vi "ToolScanTest.vi"(8 "error in (no error)":errorcluster, 11 "VISA resource name":refnum<visa-resource-name>="COM5") -> (0 "error out":errorcluster, 1 "read string 3":string, 2 "read string 2":string, 3 "read string":string, 4 "read string 6":string, 5 "Array":string[](array[string]))   [LabVIEW 2019]
panel:
  out "read string 13":string
  out "read string 12":string
  out "read string 11":string
  out "read string 10":string
  out "read string 9":string
  out "read string 8":string
  out "read string 5":string
  out "read string 4":string
  in  "stop":bool
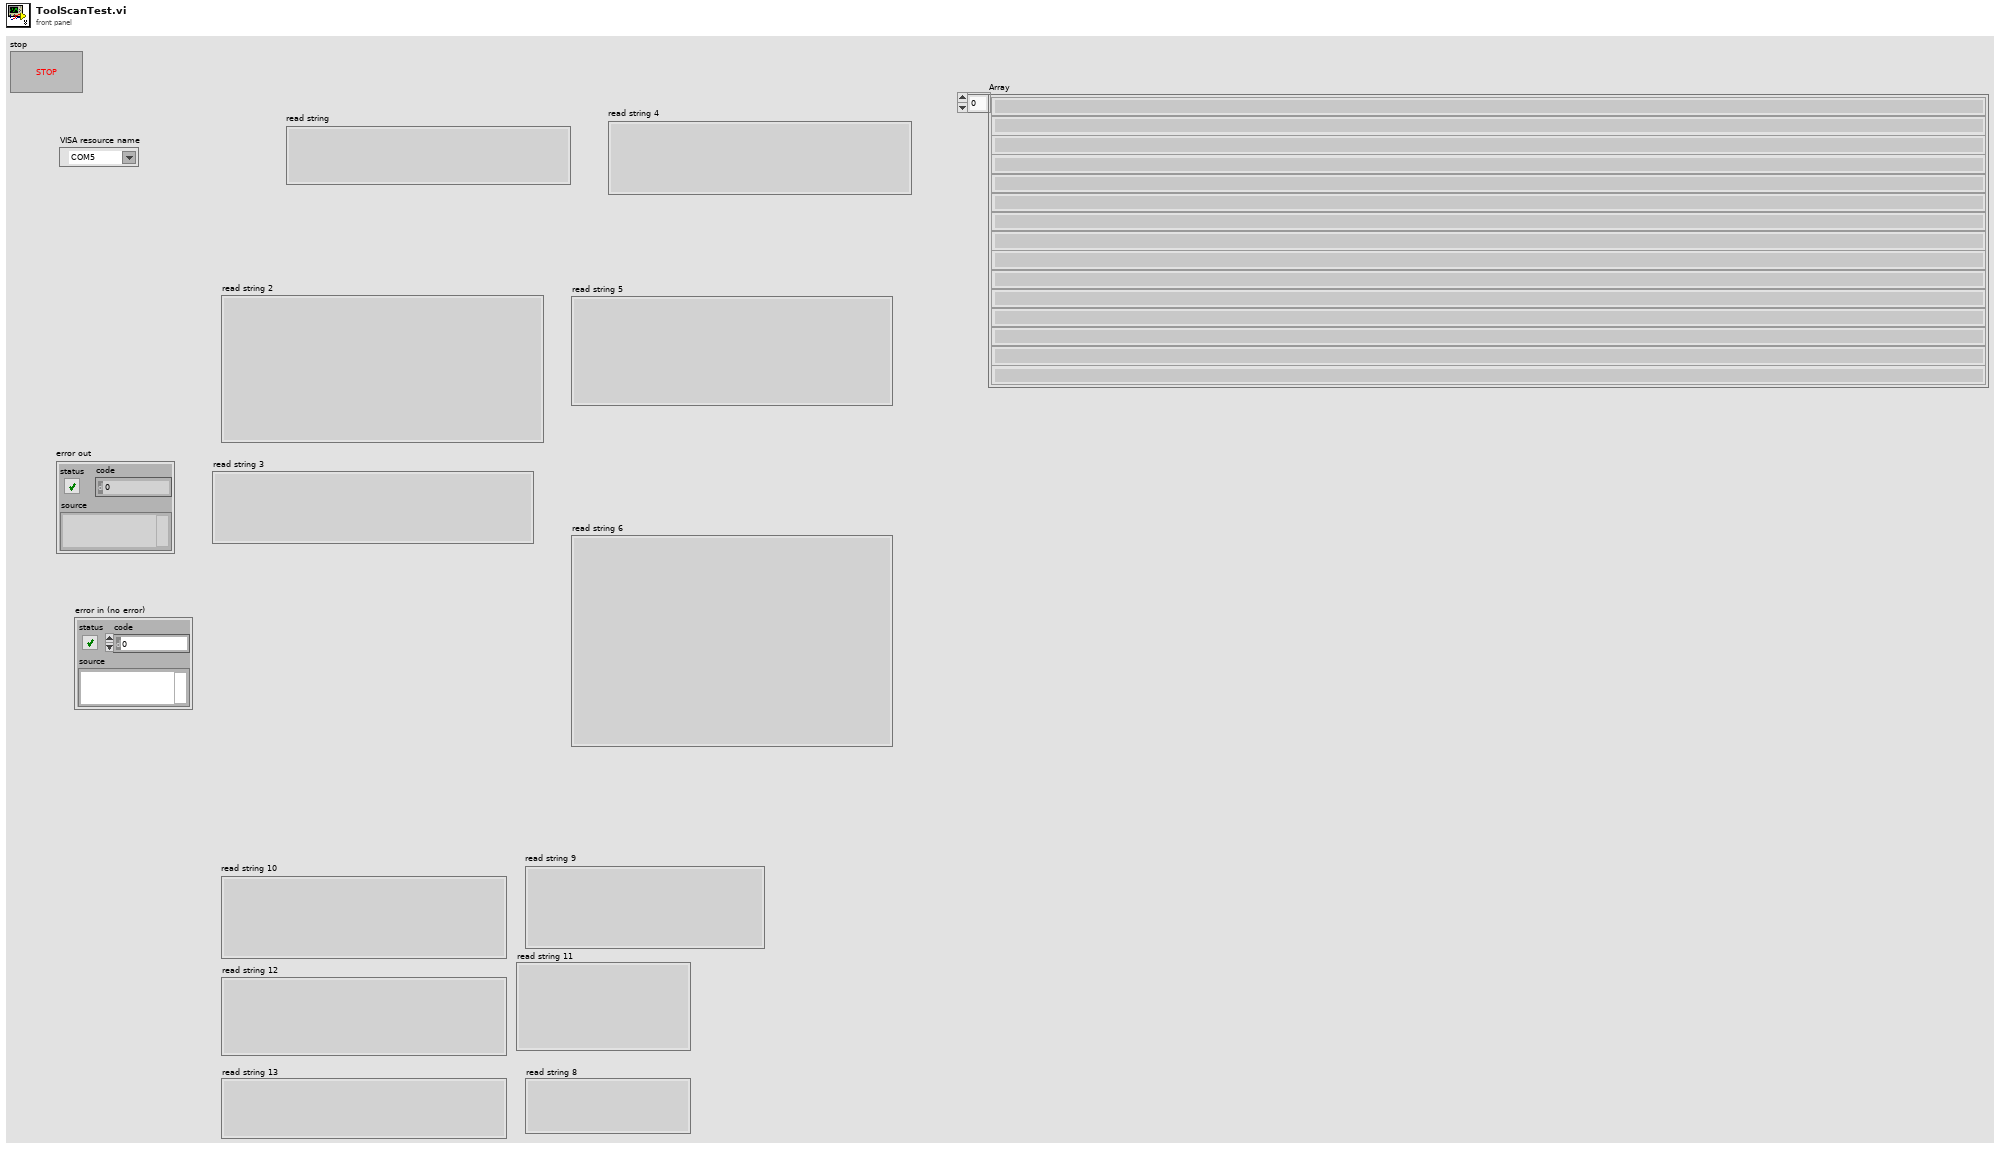
[diagram p1: front panel]
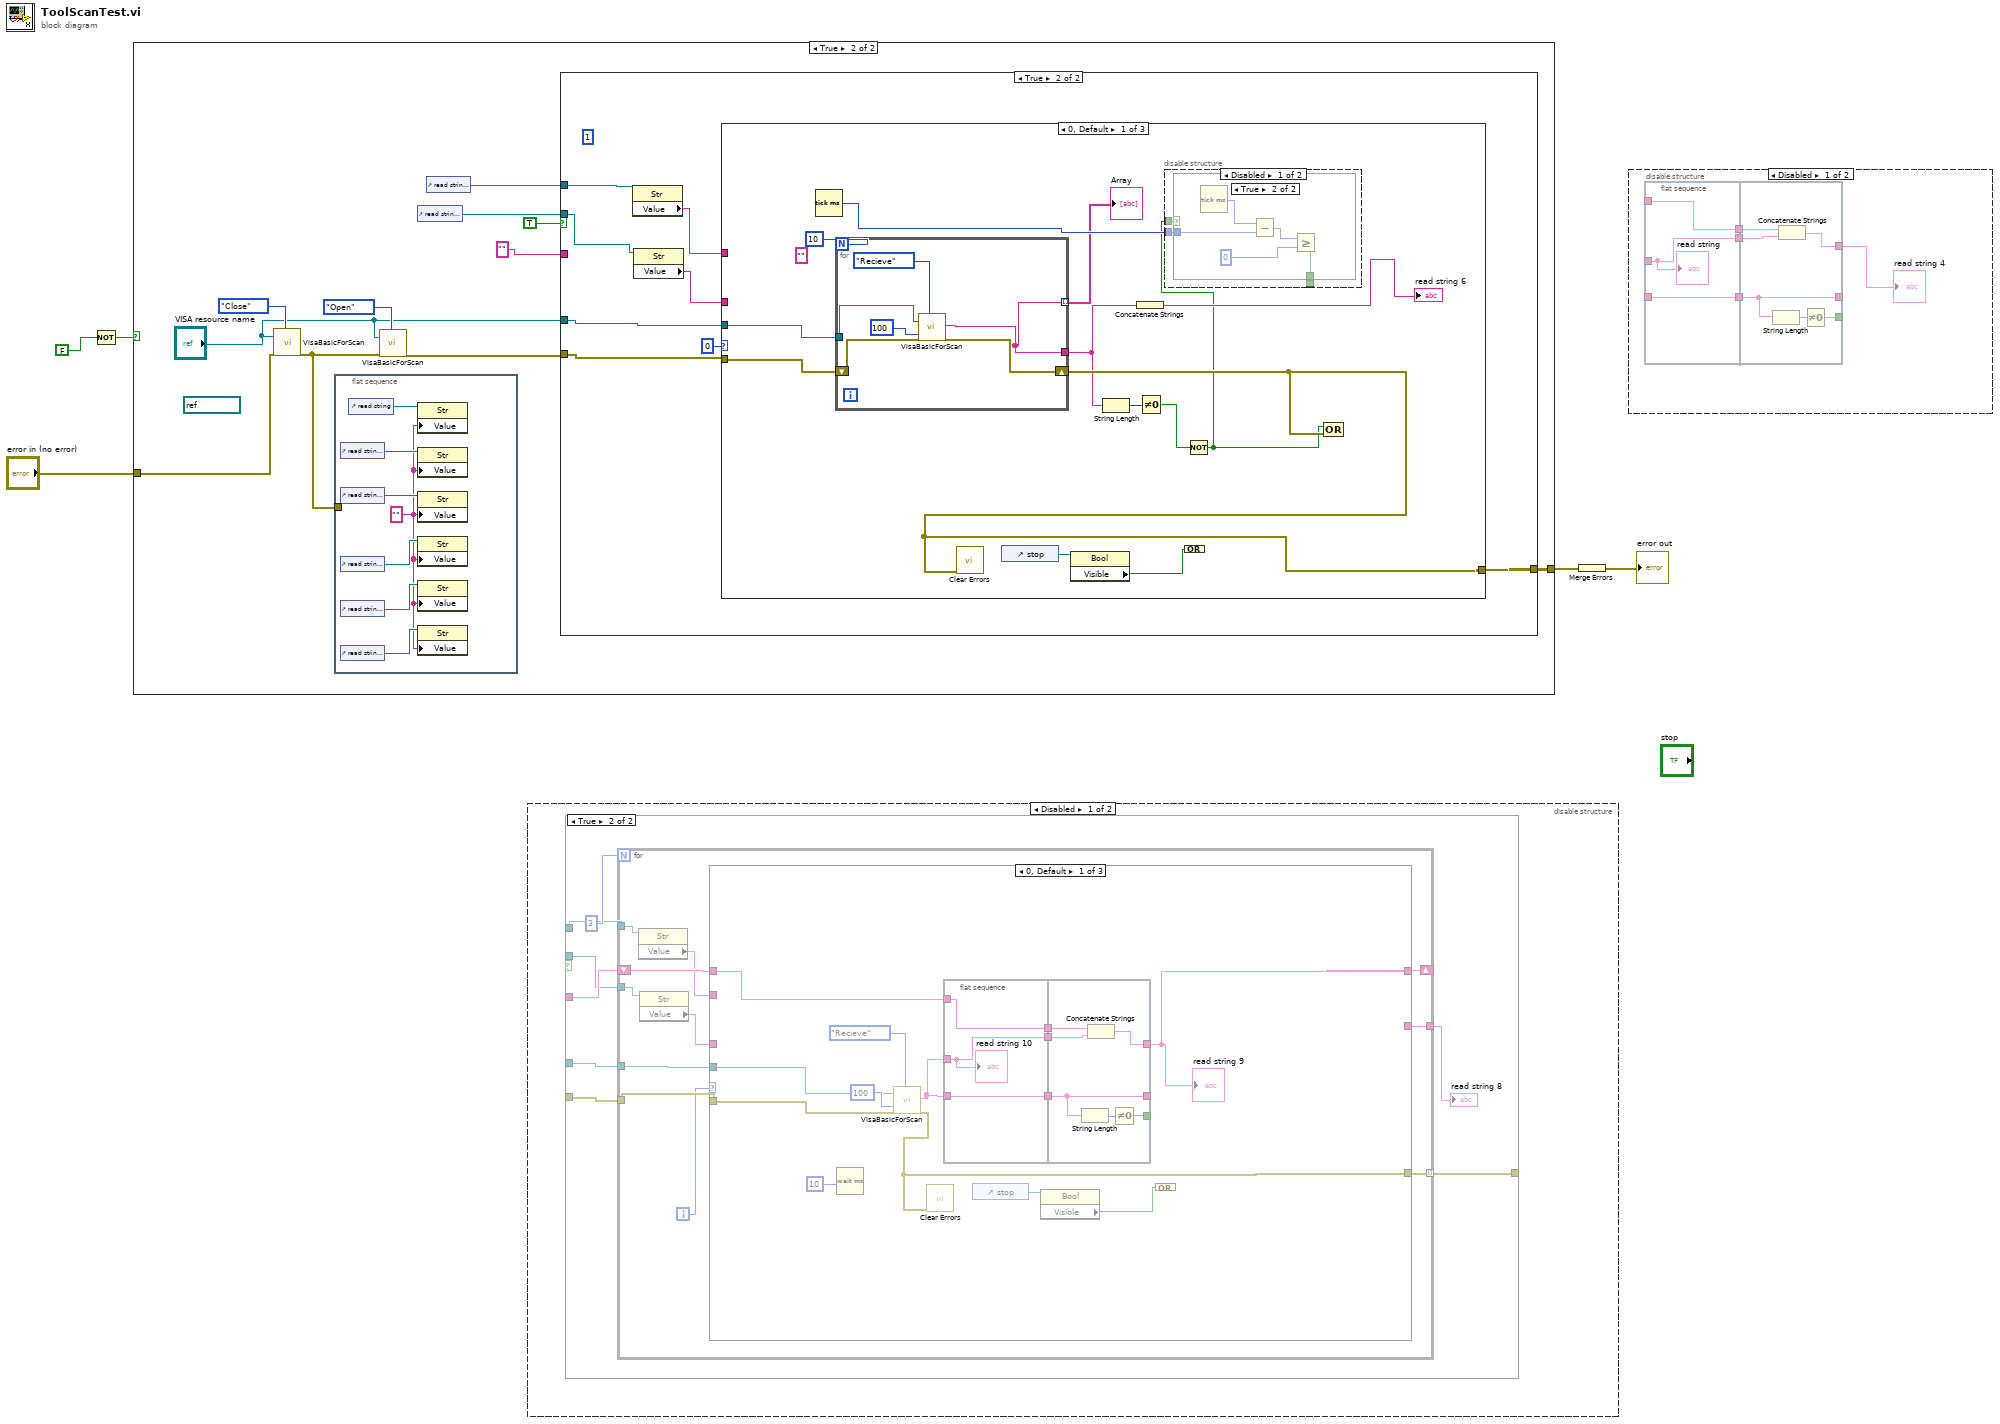
[diagram p0: block diagram]
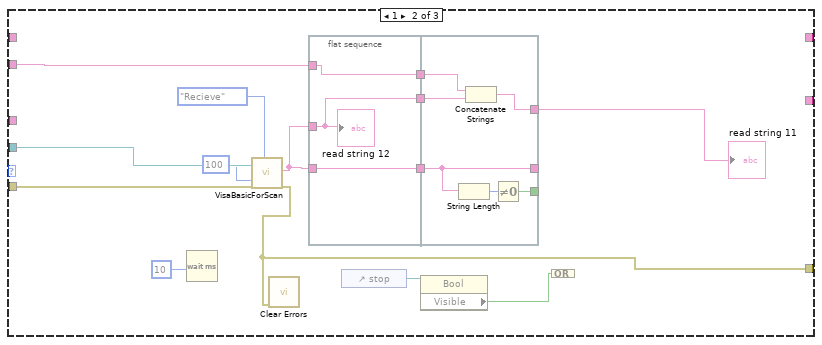
[diagram p4: hidden frame]
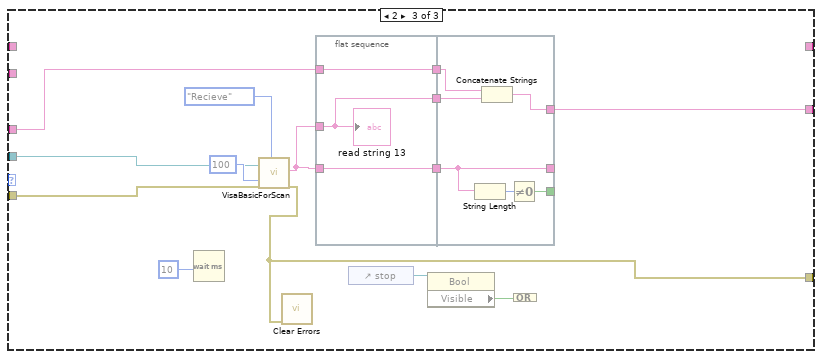
[diagram p5: hidden frame]
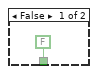
[diagram p9: hidden frame]
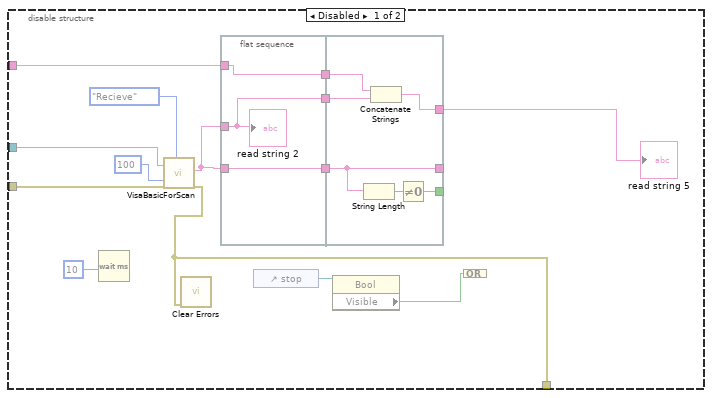
[diagram p12: hidden frame]
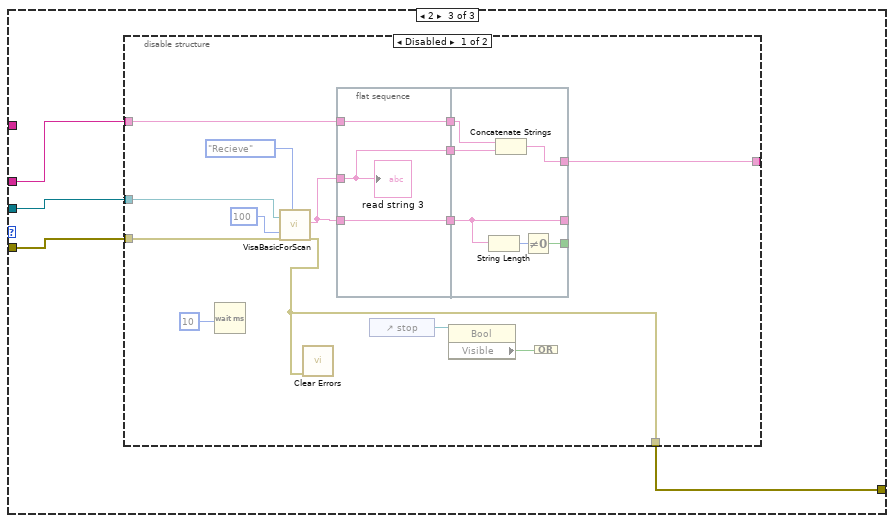
[diagram p13: hidden frame]
diagram:
  n1 = Not(x=FALSE) -> (.not. x?=w4:bool)
  n2 = case shown="True" w4 {
    tunnel: [_ w7] -> w3
    tunnel: "error in (no error)" -> [_ w6]
    frame False {
    }
    frame True {
      (unwired) refnum<visa-resource-name> "COM5" ("VISA resource name")
      n3 = call "VisaBasicForScan.vi"("VISA resource name"="VISA resource name", "error in (no error)"=w6, "VisaAction"=enum16{"Open", "Send", "Recieve", "Close"}."Close") -> ("error out"=w12:errorcluster)  [unwired: 15 in, 1 out]
      n4 = flat-sequence {
        tunnel: w12 -> [_]
        frame #0 {
          w17 = "" ("read string")
          n5 = control-ref of="read string 2"() -> (w21:refnum<vi>)
          n6 = control-ref of="read string 3"() -> (w22:refnum<vi>)
          n7 = control-ref of="read string 4"() -> (w20:refnum<vi>)
          n8 = control-ref of="read string 5"() -> (w19:refnum<vi>)
          n9 = control-ref of="read string 6"() -> (w18:refnum<vi>)
          n10 = control-ref of="read string"() -> (w23:refnum<vi>)
          n11 = property class="Str"(reference=w23, "Value"=w17) -> ()  [unwired: 1 in, 2 out]
          n12 = property class="Str"(reference=w21, "Value"=w17) -> ()  [unwired: 1 in, 2 out]
          n13 = property class="Str"(reference=w22, "Value"=w17) -> ()  [unwired: 1 in, 2 out]
          n14 = property class="Str"(reference=w20, "Value"=w17) -> ()  [unwired: 1 in, 2 out]
          n15 = property class="Str"(reference=w19, "Value"=w17) -> ()  [unwired: 1 in, 2 out]
          n16 = property class="Str"(reference=w18, "Value"=w17) -> ()  [unwired: 1 in, 2 out]
        }
      }
      n17 = call "VisaBasicForScan.vi"("VISA resource name"="VISA resource name", "error in (no error)"=w12, "VisaAction"=enum16{"Open", "Send", "Recieve", "Close"}."Open") -> ("error out"=w14:errorcluster)  [unwired: 15 in, 1 out]
      n18 = control-ref of="read string 5"() -> (w10:refnum<vi>)
      n19 = control-ref of="read string 4"() -> (w11:refnum<vi>)
      n20 = case shown="True" TRUE {
        tunnel: w14 -> [_ w31]
        tunnel: "VISA resource name" -> [_ w30]
        tunnel: "" ("read string") -> [_ _]
        tunnel: w11 -> [_ w29]
        tunnel: w10 -> [_ w28]
        tunnel: [_ w27] -> w7
        frame False {
        }
        frame True {
          (unwired) 1
          n21 = property class="Str"(reference=w29) -> ("Value"=w26:string)  [unwired: 1 in, 2 out]
          n22 = property class="Str"(reference=w28) -> ("Value"=w25:string)  [unwired: 1 in, 2 out]
          n23 = case shown="0, Default" 0 {
            tunnel: w31 -> [w41 w63 w90]
            tunnel: w30 -> [w42 w62 w91]
            tunnel: w26 -> [_ w61 _]
            tunnel: w25 -> [_ _ w89]
            tunnel: [w40 w60 w88] -> w27
            frame 0, Default {
              (unwired) "" ("read string")
              n24 = Tick Count (ms)() -> (millisecond timer value=w39:u32)
              n25 = for {
                N: 10 -> [_]
                tunnel: w42 -> [w50]
                tunnel: [w45] -> w35
                shift-right: [w48] -> w40
                shift-left: w41 -> [w49]
                tunnel: [w45] -> w32 mode=indexing
                n26 = call "VisaBasicForScan.vi"("VISA resource name"=w50, "Time(0.1)"=u32 100, "error in (no error)"=w49, "VisaAction"=enum16{"Open", "Send", "Recieve", "Close"}."Recieve") -> ("read string"=w45:string, "error out"=w48:errorcluster)  [unwired: 14 in]
              }
              "Array" <- w32
              n27 = call <vilib>:"Clear Errors.vi"("error in (no error)"=w40) -> ()  [unwired: 5 in, 2 out]
              n28 = control-ref of="stop"() -> (w44:refnum<vi>)
              n29 = property class="Bool"(reference=w44) -> ("Visible"=w43:bool)  [unwired: 1 in, 2 out]
              n30 = String Length(string=w35) -> (length=w37:i32)
              n31 = Concatenate Strings(w35) -> (→"read string 6":string)
              n32 = Not Equal To 0?(x=w37) -> (x != 0?=w36:bool)
              n33 = Not(x=w36) -> (.not. x?=w34:bool)
              n34 = disable-structure shown="Disabled" {
                disable-tunnel: w39 -> [w53 _]
                disable-tunnel: w34 -> [w52 _]
                disable-tunnel: [w51 _] -> _
                frame Disabled {
                  n35 = case shown="True" w52 {
                    tunnel: w53 -> [_ w58]
                    tunnel: [FALSE w55] -> w51
                    frame False {
                    }
                    frame True {
                      n36 = Tick Count (ms)() -> (millisecond timer value=w59:u32)
                      n37 = Subtract(x=w59, y=w58) -> (x-y=w57:u32)
                      n38 = Greater Or Equal?(x=w57, y=0) -> (x >= y?=w55:bool)
                    }
                  }
                }
                frame Enabled {
                }
              }
              n39 = Compound Arithmetic op=OR(w43) -> ()  [unwired: 1 out]
              n40 = Compound Arithmetic op=OR(w34, w40) -> ()  [unwired: 1 out]
            }
            frame 1 {
              n41 = disable-structure shown="Enabled" {
                disable-tunnel: w63 -> [w74 _]
                disable-tunnel: w62 -> [w73 _]
                disable-tunnel: w61 -> [w66 w87]
                disable-tunnel: [w64 _] -> w60
                disable-tunnel: [_ w87] -> _
                frame Disabled {
                  n42 = Wait (ms)(milliseconds to wait=10) -> ()  [unwired: 1 out]
                  n43 = call "VisaBasicForScan.vi"("VISA resource name"=w73, "Time(0.1)"=u32 100, "error in (no error)"=w74, "VisaAction"=enum16{"Open", "Send", "Recieve", "Close"}."Recieve") -> ("read string"=w70:string, "error out"=w64:errorcluster)  [unwired: 14 in]
                  n44 = call <vilib>:"Clear Errors.vi"("error in (no error)"=w64) -> ()  [unwired: 5 in, 2 out]
                  n45 = flat-sequence {
                    tunnel: w70 -> [w79]
                    tunnel: w70 -> [w80]
                    tunnel: [w80] -> w77
                    tunnel: [w78] -> w76
                    tunnel: [w79] -> w75
                    tunnel: w66 -> [w78]
                    tunnel: w77 -> [w84]
                    tunnel: [w84] -> _
                    tunnel: [w85] -> _
                    tunnel: [w83] -> w65
                    tunnel: w76 -> [w82]
                    tunnel: w75 -> [w81]
                    frame #0 {
                      "read string 2" <- w79
                    }
                    frame #1 {
                      n46 = String Length(string=w84) -> (length=w86:i32)
                      n47 = Concatenate Strings(w82, w81) -> (w83:string)
                      n48 = Not Equal To 0?(x=w86) -> (x != 0?=w85:bool)
                    }
                  }
                  n49 = control-ref of="stop"() -> (w69:refnum<vi>)
                  n50 = property class="Bool"(reference=w69) -> ("Visible"=w68:bool)  [unwired: 1 in, 2 out]
                  n51 = Compound Arithmetic op=OR(w68) -> ()  [unwired: 1 out]
                  "read string 5" <- w65
                }
                frame Enabled {
                }
              }
            }
            frame 2 {
              n52 = disable-structure shown="Disabled" {
                disable-tunnel: w91 -> [w96 _]
                disable-tunnel: w90 -> [w95 _]
                disable-tunnel: w89 -> [w94 _]
                disable-tunnel: [w93 _] -> _
                disable-tunnel: [w92 _] -> w88
                frame Disabled {
                  n53 = Wait (ms)(milliseconds to wait=10) -> ()  [unwired: 1 out]
                  n54 = call "VisaBasicForScan.vi"("VISA resource name"=w96, "Time(0.1)"=u32 100, "error in (no error)"=w95, "VisaAction"=enum16{"Open", "Send", "Recieve", "Close"}."Recieve") -> ("read string"=w102:string, "error out"=w92:errorcluster)  [unwired: 14 in]
                  n55 = call <vilib>:"Clear Errors.vi"("error in (no error)"=w92) -> ()  [unwired: 5 in, 2 out]
                  n56 = flat-sequence {
                    tunnel: w102 -> [w107]
                    tunnel: w102 -> [w108]
                    tunnel: [w108] -> w105
                    tunnel: [w107] -> w104
                    tunnel: w94 -> [w106]
                    tunnel: [w106] -> w103
                    tunnel: w105 -> [w112]
                    tunnel: [w112] -> _
                    tunnel: [w113] -> _
                    tunnel: [w111] -> w93
                    tunnel: w104 -> [w110]
                    tunnel: w103 -> [w109]
                    frame #0 {
                      "read string 3" <- w107
                    }
                    frame #1 {
                      n57 = String Length(string=w112) -> (length=w114:i32)
                      n58 = Concatenate Strings(w109, w110) -> (w111:string)
                      n59 = Not Equal To 0?(x=w114) -> (x != 0?=w113:bool)
                    }
                  }
                  n60 = control-ref of="stop"() -> (w101:refnum<vi>)
                  n61 = property class="Bool"(reference=w101) -> ("Visible"=w100:bool)  [unwired: 1 in, 2 out]
                  n62 = Compound Arithmetic op=OR(w100) -> ()  [unwired: 1 out]
                }
                frame Enabled {
                }
              }
            }
          }
        }
      }
    }
  }
  n63 = disable-structure shown="Disabled" {
    frame Disabled {
      n64 = case shown="True" {
        selector: _ -> [_ _]
        tunnel: _ -> [_ w122]
        tunnel: _ -> [_ w121]
        tunnel: _ -> [_ w120]
        tunnel: _ -> [_ w118]
        tunnel: _ -> [_ w117]
        tunnel: [_ w115] -> _
        frame False {
        }
        frame True {
          n65 = for {
            N: 3 -> [_]
            tunnel: w122 -> [w133]
            tunnel: w121 -> [w132]
            shift-right: [w129] -> _
            shift-left: w120 -> [w130]
            tunnel: w118 -> [w128]
            tunnel: w117 -> [w127]
            tunnel: [w124] -> w116
            tunnel: [w123] -> w115 mode=indexing
            i -> [w131]
            n66 = property class="Str"(reference=w128) -> ("Value"=w126:string)  [unwired: 1 in, 2 out]
            n67 = property class="Str"(reference=w127) -> ("Value"=w125:string)  [unwired: 1 in, 2 out]
            n68 = case shown="0, Default" w131 {
              tunnel: w133 -> [w139 w170 w185]
              tunnel: w132 -> [w140 w169 w186]
              tunnel: w126 -> [_ w159 _]
              tunnel: w125 -> [_ _ w183]
              tunnel: w130 -> [w136 _ _]
              tunnel: [w135 _ _] -> w129
              tunnel: [_ _ w181] -> w124
              tunnel: [w134 w157 w180] -> w123
              frame 0, Default {
                n69 = Wait (ms)(milliseconds to wait=10) -> ()  [unwired: 1 out]
                n70 = call "VisaBasicForScan.vi"("VISA resource name"=w140, "Time(0.1)"=u32 100, "error in (no error)"=w139, "VisaAction"=enum16{"Open", "Send", "Recieve", "Close"}."Recieve") -> ("read string"=w144:string, "error out"=w134:errorcluster)  [unwired: 14 in]
                n71 = call <vilib>:"Clear Errors.vi"("error in (no error)"=w134) -> ()  [unwired: 5 in, 2 out]
                n72 = flat-sequence {
                  tunnel: w144 -> [w148]
                  tunnel: w144 -> [w150]
                  tunnel: [w150] -> w147
                  tunnel: w136 -> [w149]
                  tunnel: [w149] -> w138
                  tunnel: [w148] -> w137
                  tunnel: w147 -> [w154]
                  tunnel: [w154] -> _
                  tunnel: [w155] -> _
                  tunnel: [w153] -> w135
                  tunnel: w138 -> [w152]
                  tunnel: w137 -> [w151]
                  frame #0 {
                    "read string 10" <- w148
                  }
                  frame #1 {
                    n73 = String Length(string=w154) -> (length=w156:i32)
                    n74 = Concatenate Strings(w152, w151) -> (w153:string)
                    n75 = Not Equal To 0?(x=w156) -> (x != 0?=w155:bool)
                  }
                }
                n76 = control-ref of="stop"() -> (w143:refnum<vi>)
                n77 = property class="Bool"(reference=w143) -> ("Visible"=w142:bool)  [unwired: 1 in, 2 out]
                n78 = Compound Arithmetic op=OR(w142) -> ()  [unwired: 1 out]
                "read string 9" <- w135
              }
              frame 1 {
                n79 = Wait (ms)(milliseconds to wait=10) -> ()  [unwired: 1 out]
                n80 = call "VisaBasicForScan.vi"("VISA resource name"=w169, "Time(0.1)"=u32 100, "error in (no error)"=w170, "VisaAction"=enum16{"Open", "Send", "Recieve", "Close"}."Recieve") -> ("read string"=w165:string, "error out"=w157:errorcluster)  [unwired: 14 in]
                n81 = call <vilib>:"Clear Errors.vi"("error in (no error)"=w157) -> ()  [unwired: 5 in, 2 out]
                n82 = flat-sequence {
                  tunnel: w165 -> [w172]
                  tunnel: w165 -> [w173]
                  tunnel: [w173] -> w168
                  tunnel: [w171] -> w161
                  tunnel: [w172] -> w160
                  tunnel: w159 -> [w171]
                  tunnel: w168 -> [w177]
                  tunnel: [w177] -> _
                  tunnel: [w178] -> _
                  tunnel: [w176] -> w158
                  tunnel: w161 -> [w175]
                  tunnel: w160 -> [w174]
                  frame #0 {
                    "read string 12" <- w172
                  }
                  frame #1 {
                    n83 = String Length(string=w177) -> (length=w179:i32)
                    n84 = Concatenate Strings(w175, w174) -> (w176:string)
                    n85 = Not Equal To 0?(x=w179) -> (x != 0?=w178:bool)
                  }
                }
                n86 = control-ref of="stop"() -> (w164:refnum<vi>)
                n87 = property class="Bool"(reference=w164) -> ("Visible"=w163:bool)  [unwired: 1 in, 2 out]
                n88 = Compound Arithmetic op=OR(w163) -> ()  [unwired: 1 out]
                "read string 11" <- w158
              }
              frame 2 {
                n89 = Wait (ms)(milliseconds to wait=10) -> ()  [unwired: 1 out]
                n90 = call "VisaBasicForScan.vi"("VISA resource name"=w186, "Time(0.1)"=u32 100, "error in (no error)"=w185, "VisaAction"=enum16{"Open", "Send", "Recieve", "Close"}."Recieve") -> ("read string"=w192:string, "error out"=w180:errorcluster)  [unwired: 14 in]
                n91 = call <vilib>:"Clear Errors.vi"("error in (no error)"=w180) -> ()  [unwired: 5 in, 2 out]
                n92 = flat-sequence {
                  tunnel: w192 -> [w195]
                  tunnel: w192 -> [w196]
                  tunnel: [w196] -> w193
                  tunnel: [w195] -> w184
                  tunnel: w183 -> [w194]
                  tunnel: [w194] -> w182
                  tunnel: w193 -> [w200]
                  tunnel: [w200] -> _
                  tunnel: [w201] -> _
                  tunnel: [w199] -> w181
                  tunnel: w184 -> [w198]
                  tunnel: w182 -> [w197]
                  frame #0 {
                    "read string 13" <- w195
                  }
                  frame #1 {
                    n93 = String Length(string=w200) -> (length=w202:i32)
                    n94 = Concatenate Strings(w197, w198) -> (w199:string)
                    n95 = Not Equal To 0?(x=w202) -> (x != 0?=w201:bool)
                  }
                }
                n96 = control-ref of="stop"() -> (w191:refnum<vi>)
                n97 = property class="Bool"(reference=w191) -> ("Visible"=w190:bool)  [unwired: 1 in, 2 out]
                n98 = Compound Arithmetic op=OR(w190) -> ()  [unwired: 1 out]
              }
            }
          }
          "read string 8" <- w116
        }
      }
    }
    frame Enabled {
    }
  }
  n99 = Merge Errors(w3) -> (→"error out":errorcluster)
  n100 = disable-structure shown="Disabled" {
    frame Disabled {
      n101 = flat-sequence {
        tunnel: _ -> [w207]
        tunnel: _ -> [w209]
        tunnel: [w209] -> w206
        tunnel: _ -> [w208]
        tunnel: [w208] -> w205
        tunnel: [w207] -> w204
        tunnel: w206 -> [w213]
        tunnel: [w213] -> _
        tunnel: [w214] -> _
        tunnel: [w212] -> w203
        tunnel: w205 -> [w211]
        tunnel: w204 -> [w210]
        frame #0 {
          "read string" <- w207
        }
        frame #1 {
          n102 = String Length(string=w213) -> (length=w215:i32)
          n103 = Concatenate Strings(w211, w210) -> (w212:string)
          n104 = Not Equal To 0?(x=w215) -> (x != 0?=w214:bool)
        }
      }
      "read string 4" <- w203
    }
    frame Enabled {
    }
  }
